vi "Read ExtractedData Config.vi"(8 "error in (no error)":errorcluster, 11 "MassSpectrumExtractor in":refnum<class "MassSpectrumExtractor.lvclass">) -> (0 "error out":errorcluster, 2 "Extracted Data Info":cluster{"Name":string, "Config":variant}[](array[cluster]), 3 "MassSpectrumExtractor out":refnum<class "MassSpectrumExtractor.lvclass">)   [LabVIEW 2014, in "MassSpectrumExtractor.lvclass"]
uses:
  MassSpectrumExtractor.lvclass
  AbstractExtractor1D/AbstractExtractor1D.lvclass
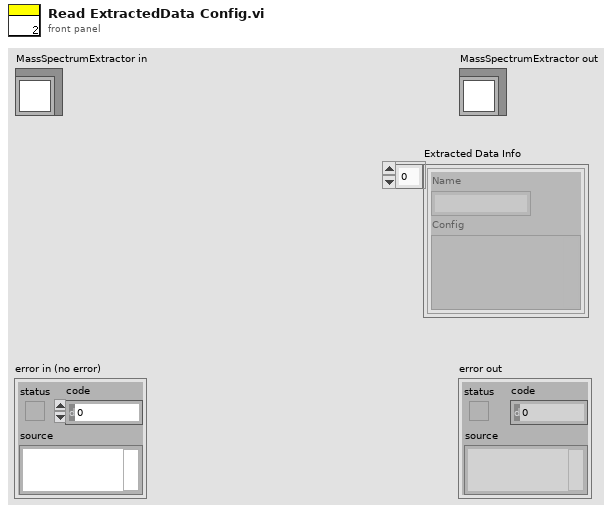
[diagram p1: front panel]
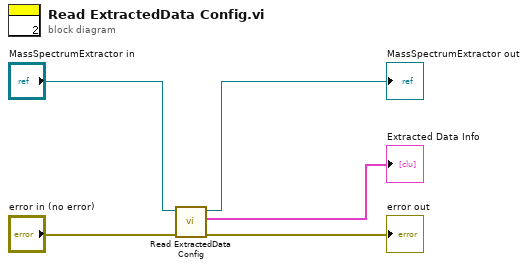
[diagram p0: block diagram]
diagram:
  n1 = call-parent "Read ExtractedData Config.vi"("error in (no error)"="error in (no error)", "AbstractExtractor in"="MassSpectrumExtractor in") -> ("error out"=→"error out":errorcluster, "Extracted Data Info"=→"Extracted Data Info":cluster{"Name":string, "Config":variant}[], "AbstractExtractor out"=→"MassSpectrumExtractor out":refnum<class "MassSpectrumExtractor.lvclass">)  [unwired: 7 in]
